vi "GetParam.vi"(8 "error in (no error)":errorcluster caption="entrée d'erreur (pas d'erreur)", 11 "TfidfTransformer.lvclass":refnum<class "TfidfTransformer.lvclass">) -> (0 "error out":errorcluster caption="sortie d'erreur", 2 "TfidfTransformer":T1={"norm"="l2", "use_idf"=TRUE, "smooth_idf"=TRUE, "sublinear_tf"=FALSE}, 3 "TfidfTransformer.lvclass":refnum<class "TfidfTransformer.lvclass">)   [LabVIEW 2020, in "TfidfTransformer.lvclass"]
doc: "Get Parameters"
uses:
  TfidfTransformer.lvclass
  TfidfTransformer.lvclass/TfidfTransformer.ctl
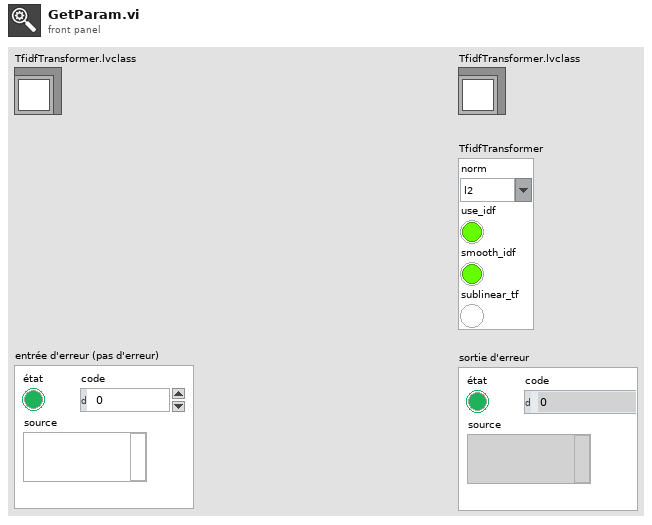
[diagram p1: front panel]
types:
  T1 = cluster{"norm":string, "use_idf":bool, "smooth_idf":bool, "sublinear_tf":bool}
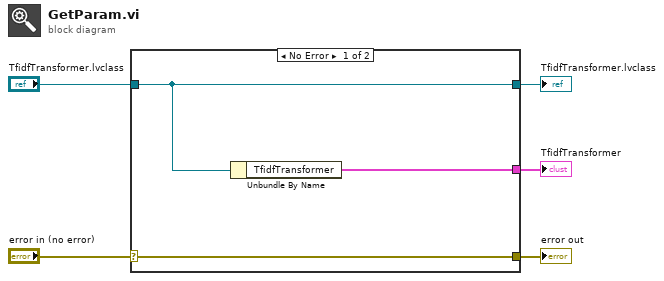
[diagram p0: block diagram]
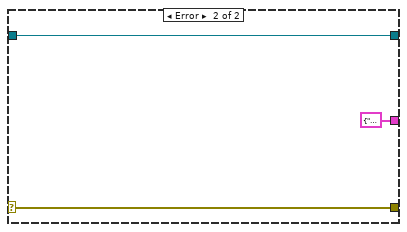
[diagram p2: hidden frame]
diagram:
  n1 = case shown="No Error" "error in (no error)" {
    selector: "error in (no error)" -> [w8 w10]
    tunnel: [w8 w10] -> w4
    tunnel: [w7 w11] -> w2
    tunnel: "TfidfTransformer.lvclass" -> [w7 w11]
    tunnel: [w6 T1 {"norm"="", "use_idf"=FALSE, "smooth_idf"=FALSE, "sublinear_tf"=FALSE} ("TfidfTransformer")] -> w1
    frame No Error {
      n2 = Unbundle By Name(w7) -> ("TfidfTransformer"=w6:T1)
    }
    frame Error {
    }
  }
  "error out" <- w4
  "TfidfTransformer.lvclass" <- w2
  "TfidfTransformer" <- w1
